vi "FTW-Container-AddOrReplace.vi"(0 "Container":refnum<class "FTW-Container.lvclass">, 5 "Value":variant, 11 "error in":errorcluster) -> (4 "Container out":refnum<class "FTW-Container.lvclass">, 6 "Replaced?":bool, 15 "error out":errorcluster)   [LabVIEW 2014, in "FTW-Container.lvclass"]
uses:
  FTW-Container.lvclass
panel:
  # "Inputs"
  # "Outputs"
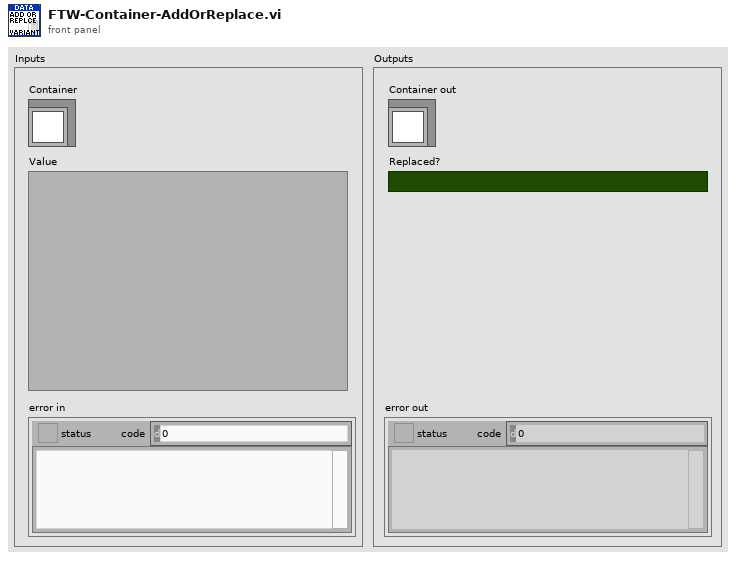
[diagram p1: front panel]
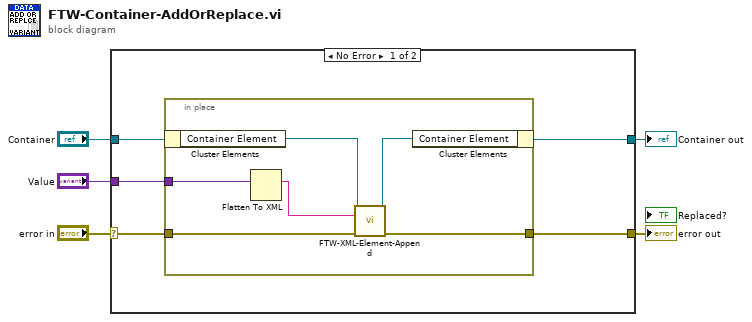
[diagram p0: block diagram]
diagram:
  n1 = case shown="No Error" "error in" {
    selector: "error in" -> [w9 w18]
    tunnel: [w8 w18] -> w5
    tunnel: "Container" -> [w10 w17]
    tunnel: [w7 w17] -> w2
    tunnel: "Value" -> [w6 _]
    frame No Error {
      n2 = in-place {
        in-place-border: w9 -> [w14]
        in-place-border: [w13] -> w8
        in-place-border: w6 -> [w12]
        n3 = in-place-cluster #1(w10) -> ("Container Element"=w16:refnum<k20>)
        n4 = Flatten To XML(anything=w12) -> (xml string=w11:string)
        n5 = call "FTW-XML-Element-Append.vi"("Parent Element"=w16, "XML Element to Append"=w11, "error in"=w14) -> ("Parent Element out"=w15:refnum<k20>, "error out"=w13:errorcluster)  [unwired: 10 in, 1 out]
        n6 = in-place-cluster #1("Container Element"=w15) -> (w7:refnum<class "FTW-Container.lvclass">)
      }
    }
    frame Error {
    }
  }
  "error out" <- w5
  "Container out" <- w2
